vi "Merge Error.vi"(10 "Error":errorcluster, 11 "jettl Queue Actor in":refnum<class "jettl Queue Actor.lvclass">) -> (3 "jettl Queue Actor out":refnum<class "jettl Queue Actor.lvclass">)   [LabVIEW 2021, in "jettl.lvlib" / "jettl Queue Actor.lvclass"]
uses:
  jettl Queue Actor.lvclass
  jettl Queue Actor.lvclass/jettl Queue Actor.ctl
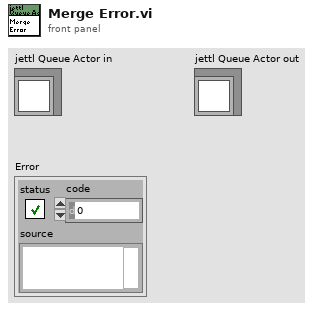
[diagram p1: front panel]
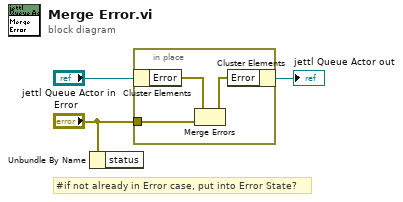
[diagram p0: block diagram]
diagram:
  # "#if not already in Error case, put into Error State?"
  n1 = Unbundle By Name("Error") -> ()  [unwired: 1 out]
  n2 = in-place {
    in-place-border: "Error" -> [w4]
    n3 = in-place-cluster #1("jettl Queue Actor in") -> ("Error"=w6:errorcluster)
    n4 = Merge Errors(w6, w4) -> (w5:errorcluster)
    n5 = in-place-cluster #1("Error"=w5) -> (→"jettl Queue Actor out":refnum<class "jettl Queue Actor.lvclass">)
  }
